vi "AutoDrive.vi"   [LabVIEW 2015]
uses:
  Common Code/Drivetrain Modes.ctl
  Common Code/Drivetrain Commands.ctl
  Robot Global Data.vi
types:
  T1 = typedef "Drivetrain Commands.ctl" = cluster{"Y Power":dbl, "Turn Power":dbl, "1st Gear?":bool, "Modes":T2, "Heading Target":dbl, "X Max Speed":dbl, "Y Max Speed":dbl, "X Min Speed":dbl, "Y Min Speed":dbl, "Y Target":dbl}
  T2 = typedef "Drivetrain Modes.ctl" = enum16{"Climb", "Manual", "Vision Targeting", "PID Distance Drive", "Hybrid"}
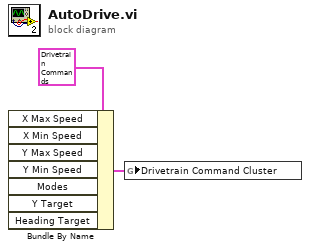
[diagram p0: block diagram]
diagram:
  n1 = Bundle By Name(cluster=T1 {"Y Power"=0.0, "Turn Power"=0.0, "1st Gear?"=FALSE, "Modes"=enum."Manual", "Heading Target"=0.0, "X Max Speed"=0.0, "Y Max Speed"=0.0, "X Min Speed"=0.0, "Y Min Speed"=0.0, "Y Target"=0.0} ("Drivetrain Command Cluster")) -> (w1:T1)  [unwired: 7 in]
  n2 = global write "Robot Global Data.vi" "Drivetrain Command Cluster"(w1) -> ()
